vi "niRFUtil WFM Sort Array (real array).vi"(2 "Sort Method":enum16{"Ascending", "Descending"}(ring), 3 "Data In":T1 min=0 max=127 format="%.2f") -> (0 "Sorted Order":i32[](array[numeric]) min=0 max=127, 1 "Sorted Data Out":T1 min=0 max=127 format="%.2f")   [LabVIEW 2015, in "niRFUtil.lvlib"]
doc: "(c) Copyright 2006, National Instruments, Inc. This VI may not be duplicated, sold, or distributed without written consent from National Instruments."
uses:
  niRFUtil.lvlib
  Includes/niRFUtil INC Real Array.ctl
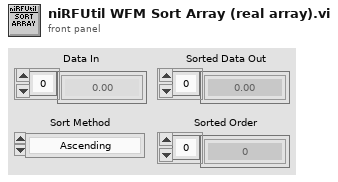
[diagram p1: front panel]
types:
  T1 = typedef "niRFUtil.lvlib/niRFUtil INC Real Array.ctl" = sgl[]
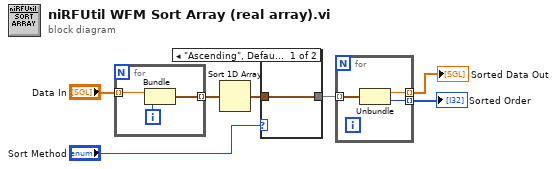
[diagram p0: block diagram]
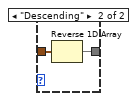
[diagram p2: hidden frame]
diagram:
  n1 = for {
    tunnel: [w10] -> w5 mode=indexing
    tunnel: "Data In" -> [w9] mode=indexing
    i -> [w8]
    n2 = Bundle("Numeric"=w9, w8) -> (w10:cluster{"Numeric":sgl, i32})  [unwired: 1 in]
  }
  n3 = Sort 1D Array(array=w5) -> (sorted array=w4:cluster{"Numeric":sgl, i32}[])
  n4 = case shown="\"Ascending\", Default" "Sort Method" {
    tunnel: w4 -> [w11 w13]
    tunnel: [w11 w12] -> w3
    frame "Ascending", Default {
    }
    frame "Descending" {
      n5 = Reverse 1D Array(array=w13) -> (reversed array=w12:cluster{"Numeric":sgl, i32}[])
    }
  }
  n6 = for {
    tunnel: w3 -> [w16] mode=indexing
    tunnel: [w15] -> w6 mode=indexing
    tunnel: [w14] -> w1 mode=indexing
    n7 = Unbundle(w16) -> ("Numeric"=w15:sgl, w14:i32)
  }
  "Sorted Data Out" <- w6
  "Sorted Order" <- w1
